vi "example_01_download.vi"() -> ()   [LabVIEW 2015, in "lv-dropbox.lvlib" / "v2.lvlib"]
uses:
  v2.lvlib
  private/_controls/http_configuration.ctl
  public/advanced/download-file.vi
  lv-dropbox.lvlib
panel:
  in  "target_directory":path=path "" caption="start path"
  in  "configuration":T1
  in  "authorization":string
  out "error out":errorcluster
  in  "dropbox_path":string
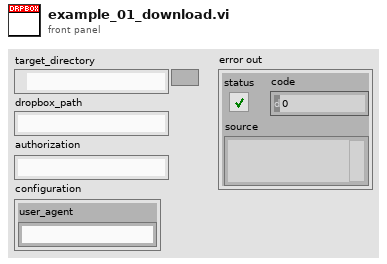
[diagram p1: front panel]
types:
  T1 = typedef "lv-dropbox.lvlib/http_configuration.ctl" = cluster{"user_agent":string}
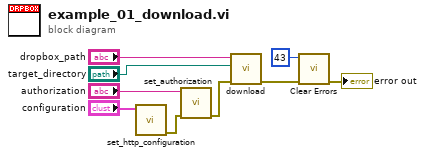
[diagram p0: block diagram]
diagram:
  n1 = call "set_http_configuration.vi"("configuration"="configuration") -> ("error out"=w3:errorcluster)  [unwired: 10 in]
  n2 = call "set_authorization.vi"("error in (no error)"=w3, "authorization"="authorization") -> ("error out"=w1:errorcluster)  [unwired: 9 in]
  n3 = call-poly "download.vi"("error in (no error)"=w1, "target_path"="target_directory", "path"="dropbox_path") -> ("error out"=w8:errorcluster)  [unwired: 8 in]
  n4 = call <vilib>:"Clear Errors.vi"("error in (no error)"=w8, "specific error code to clear (0: all)"=43) -> ("error out"=→"error out":errorcluster)  [unwired: 4 in, 1 out]
